vi "Sensor_Reads.vi"() -> ()   [LabVIEW 2019]
uses:
  M14 Hardware/Flywheel/M14_Flywheel_Hardware_Globals.vi
  <vilib>/Rock Robotics/WPI/ThirdParty/Phoenix-LabVIEW/Motor Controller/Get/CTRE_Phoenix_MotorController_GetSelectedSensorData.vi
  Sensor_Values.vi
  M14 Hardware/Drive/M14_Drive_Hardware_Globals.vi
  M14 Hardware/Spindexer/M14_Hardware_Spindexer_Globals.vi
  M14 Hardware/New Magazine/New_Magazine_Hardware_Globals.vi
  M14 Hardware/Turret/M14 Turret_Hardware_Globals.vi
  M14 Hardware/Control Panel/M14_Control_Panel_Globals.vi
  M14 Hardware/Sensors/IMU/M14_IMU_Hardware_Globals.vi
  M14 Hardware/Sensors/IRs & Limits/M14_IR&Limits_Hardware_Globals.vi
  M14 Hardware/Cowl/M14_Cowl_Hardware_Globals.vi
  <vilib>/Rock Robotics/Network Tables/NT Read Number.vi
  <vilib>/Rock Robotics/WPI/ThirdParty/Phoenix-LabVIEW/Pigeon IMU/CTRE_PigeonIMU_GetYPR.vi
panel:
  in  "ball_detected_threshold(ms)":u32
  out "Y_Position(Feet)":dbl
  out "X_Position(Feet)":dbl
  out "Right_Drive_Position(feet)":dbl
  out "Left_Drive_Position(feet)":dbl
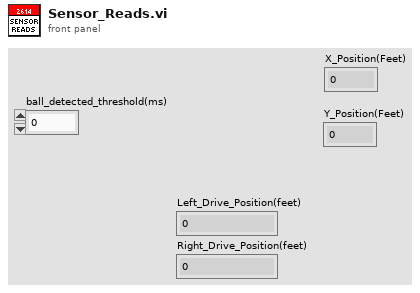
[diagram p1: front panel]
types:
  T1 = typedef "WPI_MotorControlDeviceRef.ctl" = cluster{"DeviceStatus":errorcluster, "Type":T2, "PWM":cluster{"PWM Channel":T3, "DeadBand":T4}, "CAN":cluster{"Device Number":u8, "SetOutput VI Ref":variant, "GetOutput VI Ref":variant, "Enable VI Ref":variant, "Disable VI Ref":variant, "Data":variant}, "Invert":bool, "DIO PWM":cluster{"PWM \"Enable\" Channel":T3, "DIOChannel":T5, "PWM Rate":dbl}}
  T2 = typedef "WPI_MotorControlType.ctl" = enum16{"PWM", "CAN", "DIO PWM"}
  T3 = typedef "FPGA_DIOPWMChannel.ctl" = enum8{"PWM 0", "PWM 1", "PWM 2", "PWM 3", "PWM 4", "PWM 5", "PWM 6", "PWM 7", "PWM 8", "PWM 9", "PWM MXP 0", "PWM MXP 1", "PWM MXP 2", "PWM MXP 3", "PWM MXP 4", "PWM MXP 5", "PWM MXP 6", "PWM MXP 7", "PWM MXP 8", "PWM MXP 9", "Invalid"}
  T4 = typedef "WPI_PWMDeadband.ctl" = cluster{"Name":string, "maxPositivePwm":i32, "minPositivePwm":i32, "centerPwm":i32, "maxNegativePwm":i32, "minNegativePwm":i32, "angularRange":u16}
  T5 = typedef "FPGA_DIOChannel.ctl" = enum8{"DIO 0", "DIO 1", "DIO 2", "DIO 3", "DIO 4", "DIO 5", "DIO 6", "DIO 7", "DIO 8", "DIO 9", "DIO MXP 0", "DIO MXP 1", "DIO MXP 2", "DIO MXP 3", "DIO MXP 4", "DIO MXP 5", "DIO MXP 6", "DIO MXP 7", "DIO MXP 8", "DIO MXP 9", "DIO MXP 10", "DIO MXP 11", "DIO MXP 12", "DIO MXP 13", "DIO MXP 14", "DIO MXP 15", "SPI Port CS1", "SPI Port CS2", "SPI Port CS3", "SPI Port MISO", "SPI Port MOSI", "Invalid"}
  T6 = typedef "CTRE_PigeonIMU_DeviceRef.ctl" = cluster{"DeviceStatus":errorcluster, "Device Number":u8, "Type":T7, "Device ID":u32, "Handle":u64, "UsageFrame":u32, "Library Path":path}
  T7 = typedef "CTRE_PigeonIMU_ConnectionType.ctl" = u32
  T8 = typedef "WPI_DigitalInputDevRef.ctl" = cluster{"DevStatus":errorcluster, "DIO Channel":T5}
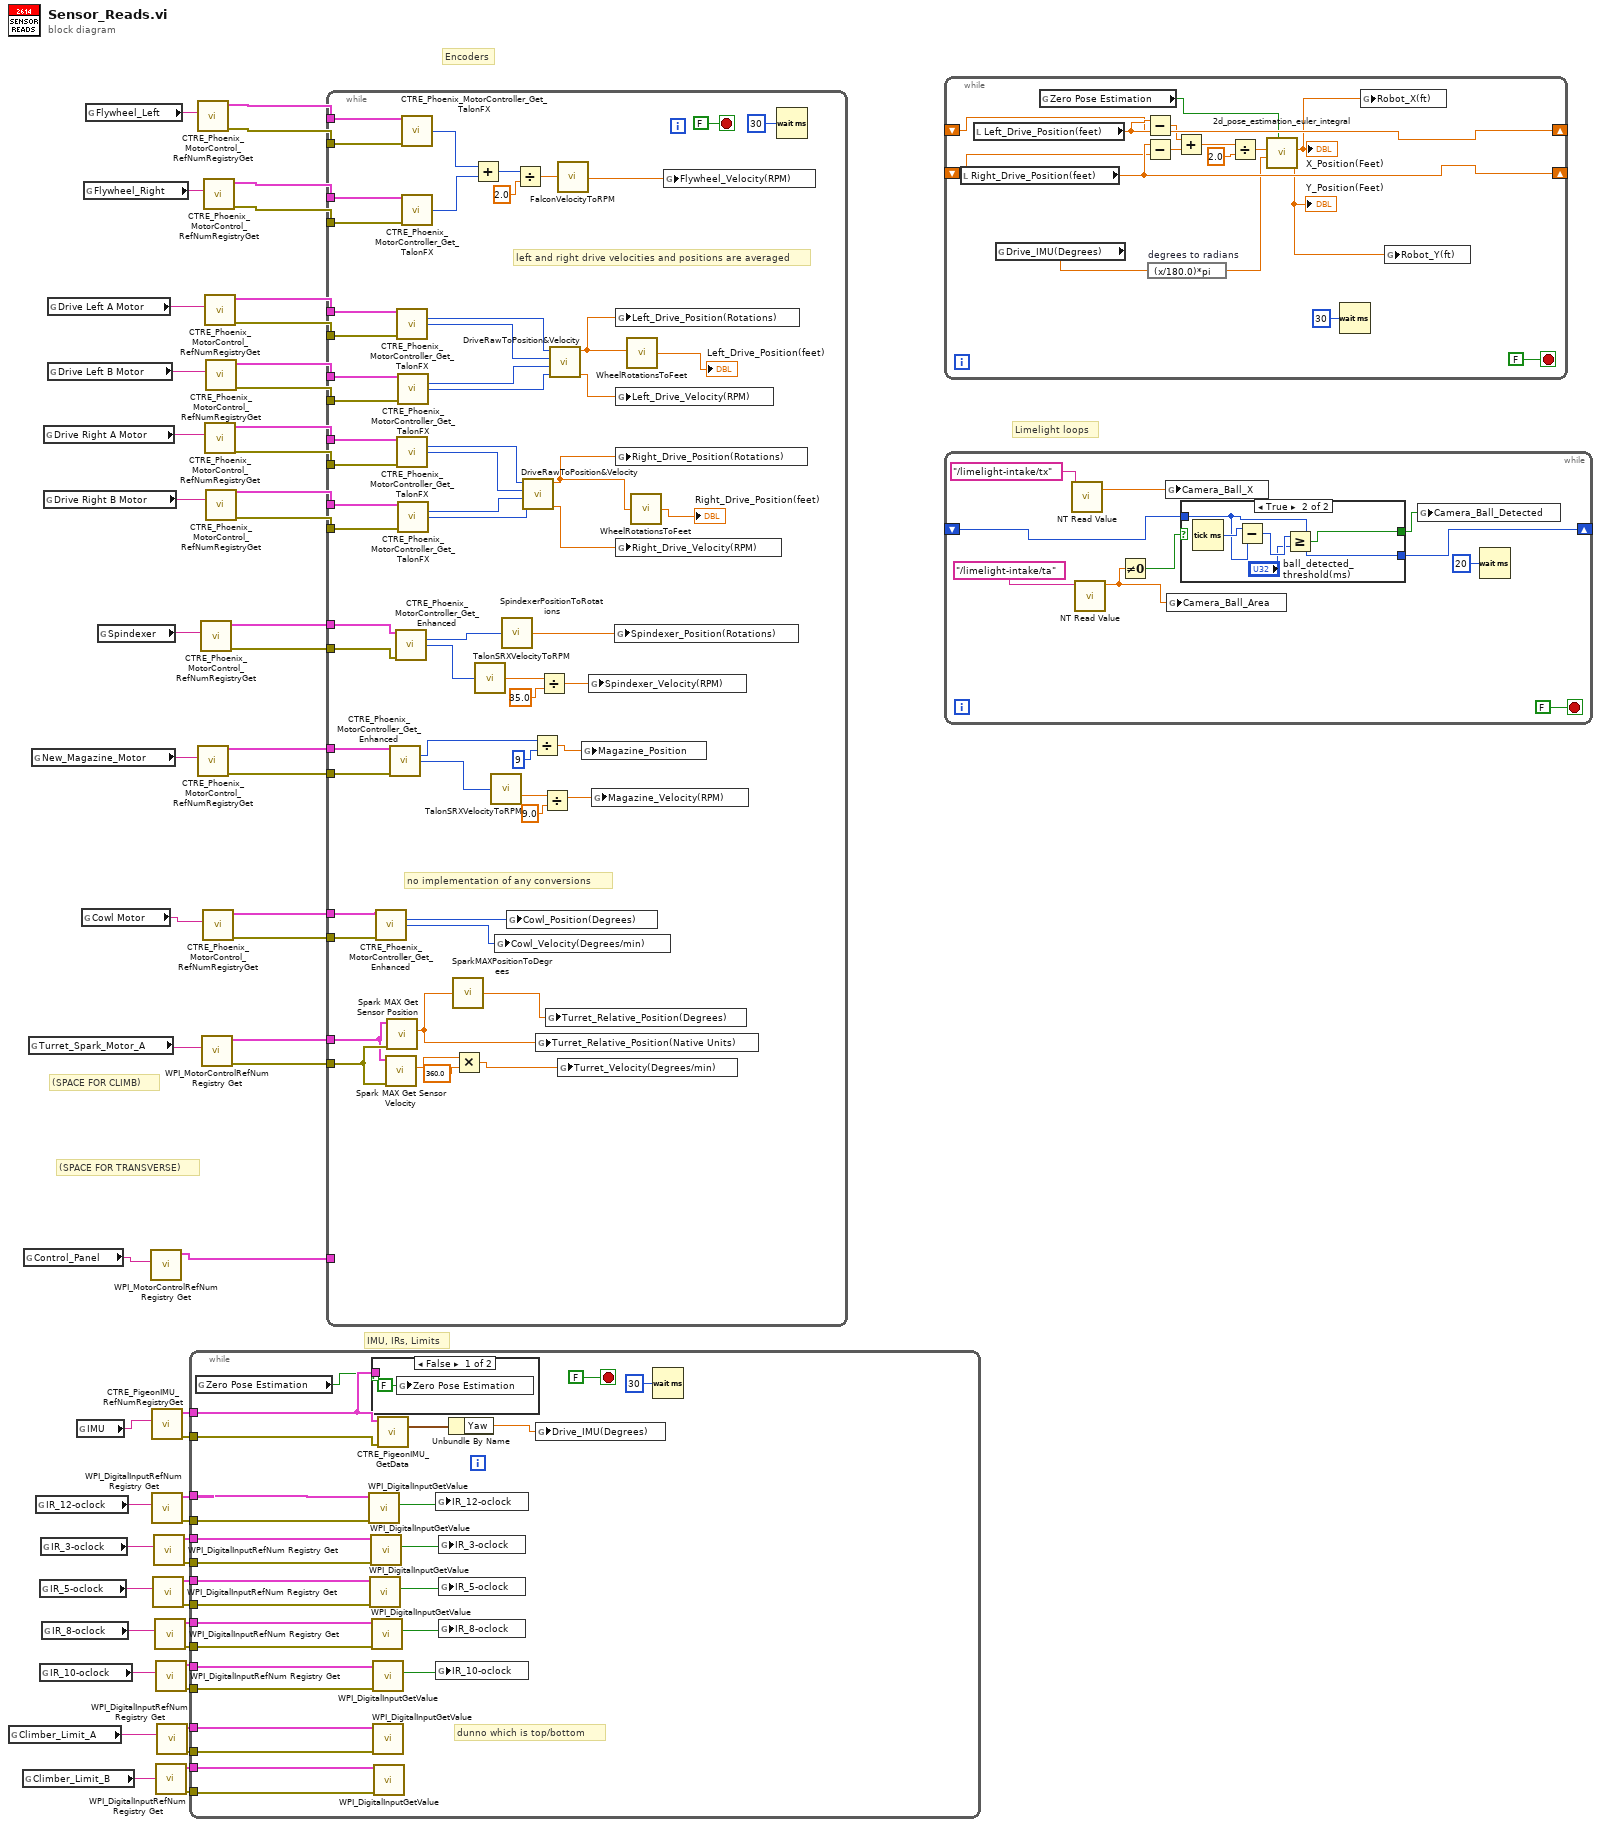
[diagram p0: block diagram]
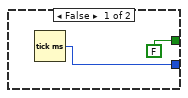
[diagram p2: hidden frame]
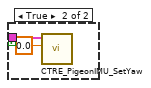
[diagram p3: hidden frame]
diagram:
  # "Limelight loops"
  # "IMU, IRs, Limits"
  # "(SPACE FOR TRANSVERSE)"
  # "(SPACE FOR CLIMB)"
  # "Encoders"
  n1 = global read "M14_IR&Limits_Hardware_Globals.vi" "Climber_Limit_A"() -> (w9:string)
  n2 = global read "M14_IR&Limits_Hardware_Globals.vi" "Climber_Limit_B"() -> (w8:string)
  n3 = global read "M14_Control_Panel_Globals.vi" "Control_Panel"() -> (w36:string)
  n4 = global read "M14 Turret_Hardware_Globals.vi" "Turret_Spark_Motor_A"() -> (w38:string)
  n5 = global read "New_Magazine_Hardware_Globals.vi" "New_Magazine_Motor"() -> (w40:string)
  n6 = global read "M14_IR&Limits_Hardware_Globals.vi" "IR_12-oclock"() -> (w22:string)
  n7 = global read "M14_IR&Limits_Hardware_Globals.vi" "IR_5-oclock"() -> (w16:string)
  n8 = global read "M14_IR&Limits_Hardware_Globals.vi" "IR_10-oclock"() -> (w10:string)
  n9 = global read "M14_IR&Limits_Hardware_Globals.vi" "IR_3-oclock"() -> (w21:string)
  n10 = global read "M14_IR&Limits_Hardware_Globals.vi" "IR_8-oclock"() -> (w15:string)
  n11 = global read "M14_Drive_Hardware_Globals.vi" "Drive Right A Motor"() -> (w43:string)
  n12 = global read "M14_Drive_Hardware_Globals.vi" "Drive Right B Motor"() -> (w46:string)
  n13 = global read "M14_Drive_Hardware_Globals.vi" "Drive Left A Motor"() -> (w50:string)
  n14 = global read "M14_Drive_Hardware_Globals.vi" "Drive Left B Motor"() -> (w47:string)
  n15 = global read "M14_IMU_Hardware_Globals.vi" "IMU"() -> (w34:string)
  n16 = global read "M14_Cowl_Hardware_Globals.vi" "Cowl Motor"() -> (w3:string)
  n17 = global read "M14_Flywheel_Hardware_Globals.vi" "Flywheel_Right"() -> (w55:string)
  n18 = global read "M14_Flywheel_Hardware_Globals.vi" "Flywheel_Left"() -> (w56:string)
  n19 = global read "M14_Hardware_Spindexer_Globals.vi" "Spindexer"() -> (w42:string)
  n20 = call <vilib>:"WPI_MotorControlRefNum Registry Get.vi"("refnum name"=w36) -> ("MotorControlDevRef"=w35:T1)  [unwired: 9 in, 1 out]
  n21 = call <vilib>:"CTRE_PigeonIMU_RefNumRegistryGet.vi"("refnum name"=w34) -> ("error out"=w25:errorcluster, "PigeonIMUDevRef"=w33:T6)  [unwired: 9 in]
  n22 = call <vilib>:"WPI_DigitalInputRefNum Registry Get.vi"("refnum name"=w22) -> ("error out"=w23:errorcluster, "DigitalInputDevRef"=w24:T8)  [unwired: 9 in]
  n23 = call <vilib>:"WPI_DigitalInputRefNum Registry Get.vi"("refnum name"=w16) -> ("error out"=w17:errorcluster, "DigitalInputDevRef"=w18:T8)  [unwired: 9 in]
  n24 = call <vilib>:"WPI_DigitalInputRefNum Registry Get.vi"("refnum name"=w21) -> ("error out"=w20:errorcluster, "DigitalInputDevRef"=w19:T8)  [unwired: 9 in]
  n25 = call <vilib>:"WPI_DigitalInputRefNum Registry Get.vi"("refnum name"=w15) -> ("error out"=w14:errorcluster, "DigitalInputDevRef"=w13:T8)  [unwired: 9 in]
  n26 = call <vilib>:"WPI_DigitalInputRefNum Registry Get.vi"("refnum name"=w10) -> ("error out"=w11:errorcluster, "DigitalInputDevRef"=w12:T8)  [unwired: 9 in]
  n27 = call <vilib>:"WPI_DigitalInputRefNum Registry Get.vi"("refnum name"=w8) -> ("error out"=w4:errorcluster, "DigitalInputDevRef"=w5:T8)  [unwired: 9 in]
  n28 = call <vilib>:"WPI_DigitalInputRefNum Registry Get.vi"("refnum name"=w9) -> ("error out"=w6:errorcluster, "DigitalInputDevRef"=w7:T8)  [unwired: 9 in]
  n29 = while {
    tunnel: w33 -> [w58]
    tunnel: w25 -> [w81]
    tunnel: w24 -> [w78]
    tunnel: w23 -> [w77]
    tunnel: w19 -> [w75]
    tunnel: w20 -> [w76]
    tunnel: w18 -> [w74]
    tunnel: w17 -> [w73]
    tunnel: w13 -> [w71]
    tunnel: w14 -> [w72]
    tunnel: w12 -> [w70]
    tunnel: w11 -> [w69]
    tunnel: w7 -> [w63]
    tunnel: w6 -> [w62]
    tunnel: w5 -> [w61]
    tunnel: w4 -> [w60]
    stop <- FALSE stop-if-true
    # "dunno which is top/bottom"
    n30 = global read "Sensor_Values.vi" "Zero Pose Estimation"() -> (w57:bool)
    n31 = call <vilib>:"WPI_DigitalInputGetValue.vi"("error in (no error)"=w77, "DigitalInputDevRef"=w78) -> ("Value"=w68:bool)  [unwired: 7 in, 2 out]
    n32 = call <vilib>:"WPI_DigitalInputGetValue.vi"("error in (no error)"=w73, "DigitalInputDevRef"=w74) -> ("Value"=w66:bool)  [unwired: 7 in, 2 out]
    n33 = call <vilib>:"WPI_DigitalInputGetValue.vi"("error in (no error)"=w76, "DigitalInputDevRef"=w75) -> ("Value"=w67:bool)  [unwired: 7 in, 2 out]
    n34 = case shown="False" w57 {
      tunnel: w58 -> [_ w85]
      frame False {
        n35 = global write "Sensor_Values.vi" "Zero Pose Estimation"(FALSE ("Zero Pose Estimation")) -> ()
      }
      frame True {
        n36 = call <vilib>:"CTRE_PigeonIMU_SetYaw.vi"("Value"=0.0, "PigeonIMUDevRef"=w85) -> ()  [unwired: 8 in, 2 out]
      }
    }
    n37 = call <vilib>:"WPI_DigitalInputGetValue.vi"("error in (no error)"=w72, "DigitalInputDevRef"=w71) -> ("Value"=w65:bool)  [unwired: 7 in, 2 out]
    n38 = call <vilib>:"WPI_DigitalInputGetValue.vi"("error in (no error)"=w69, "DigitalInputDevRef"=w70) -> ("Value"=w64:bool)  [unwired: 7 in, 2 out]
    n39 = call <vilib>:"WPI_DigitalInputGetValue.vi"("error in (no error)"=w62, "DigitalInputDevRef"=w63) -> ()  [unwired: 7 in, 3 out]
    n40 = call <vilib>:"WPI_DigitalInputGetValue.vi"("error in (no error)"=w60, "DigitalInputDevRef"=w61) -> ()  [unwired: 7 in, 3 out]
    n41 = call-poly <vilib>:"CTRE_PigeonIMU_GetData.vi"("error in (no error)"=w81, "PigeonIMUDevRef"=w58) -> ("Yaw Pitch Roll"=w80:cluster{"Yaw":dbl, "Pitch":dbl, "Roll":dbl})  [unwired: 7 in, 2 out]
    n42 = global write "Sensor_Values.vi" "IR_12-oclock"(w68) -> ()
    n43 = global write "Sensor_Values.vi" "IR_10-oclock"(w64) -> ()
    n44 = global write "Sensor_Values.vi" "IR_3-oclock"(w67) -> ()
    n45 = global write "Sensor_Values.vi" "IR_5-oclock"(w66) -> ()
    n46 = global write "Sensor_Values.vi" "IR_8-oclock"(w65) -> ()
    n47 = Unbundle By Name(w80) -> ("Yaw"=w59:dbl)
    n48 = global write "Sensor_Values.vi" "Drive_IMU(Degrees)"(w59) -> ()
    n49 = Wait (ms)(milliseconds to wait=u32 30) -> ()  [unwired: 1 out]
  }
  n50 = call <vilib>:"CTRE_Phoenix_MotorControl_RefNumRegistryGet.vi"("refnum name"=w56) -> ("error out"=w53:errorcluster, "PhoenixMotorControlDevRef"=w54:T1)  [unwired: 9 in]
  n51 = call <vilib>:"CTRE_Phoenix_MotorControl_RefNumRegistryGet.vi"("refnum name"=w40) -> ("error out"=w27:errorcluster, "PhoenixMotorControlDevRef"=w39:T1)  [unwired: 9 in]
  n52 = call <vilib>:"CTRE_Phoenix_MotorControl_RefNumRegistryGet.vi"("refnum name"=w42) -> ("error out"=w28:errorcluster, "PhoenixMotorControlDevRef"=w41:T1)  [unwired: 9 in]
  n53 = call <vilib>:"WPI_MotorControlRefNum Registry Get.vi"("refnum name"=w38) -> ("error out"=w26:errorcluster, "MotorControlDevRef"=w37:T1)  [unwired: 9 in]
  n54 = call <vilib>:"CTRE_Phoenix_MotorControl_RefNumRegistryGet.vi"("refnum name"=w3) -> ("error out"=w1:errorcluster, "PhoenixMotorControlDevRef"=w2:T1)  [unwired: 9 in]
  n55 = call <vilib>:"CTRE_Phoenix_MotorControl_RefNumRegistryGet.vi"("refnum name"=w55) -> ("error out"=w51:errorcluster, "PhoenixMotorControlDevRef"=w52:T1)  [unwired: 9 in]
  n56 = call <vilib>:"CTRE_Phoenix_MotorControl_RefNumRegistryGet.vi"("refnum name"=w50) -> ("error out"=w32:errorcluster, "PhoenixMotorControlDevRef"=w49:T1)  [unwired: 9 in]
  n57 = call <vilib>:"CTRE_Phoenix_MotorControl_RefNumRegistryGet.vi"("refnum name"=w43) -> ("error out"=w30:errorcluster, "PhoenixMotorControlDevRef"=w44:T1)  [unwired: 9 in]
  n58 = call <vilib>:"CTRE_Phoenix_MotorControl_RefNumRegistryGet.vi"("refnum name"=w47) -> ("error out"=w31:errorcluster, "PhoenixMotorControlDevRef"=w48:T1)  [unwired: 9 in]
  n59 = call <vilib>:"CTRE_Phoenix_MotorControl_RefNumRegistryGet.vi"("refnum name"=w46) -> ("error out"=w29:errorcluster, "PhoenixMotorControlDevRef"=w45:T1)  [unwired: 9 in]
  n60 = while {
    tunnel: w54 -> [w145]
    tunnel: w53 -> [w144]
    tunnel: w52 -> [w143]
    tunnel: w51 -> [w142]
    tunnel: w49 -> [w141]
    tunnel: w48 -> [w140]
    tunnel: w44 -> [w138]
    tunnel: w45 -> [w139]
    tunnel: w41 -> [w128]
    tunnel: w39 -> [w125]
    tunnel: w37 -> [w106]
    tunnel: w35 -> [_]
    tunnel: w32 -> [w113]
    tunnel: w31 -> [w112]
    tunnel: w30 -> [w111]
    tunnel: w29 -> [w110]
    tunnel: w28 -> [w109]
    tunnel: w27 -> [w108]
    tunnel: w26 -> [w107]
    tunnel: w2 -> [w89]
    tunnel: w1 -> [w88]
    stop <- FALSE stop-if-true
    # "no implementation of any conversions"
    # "left and right drive velocities and positions are averaged"
    n61 = call-poly <vilib>:"CTRE_Phoenix_MotorController_Get_Enhanced.vi"("PhoenixMotorControlDevRef"=w89, "error in"=w88) -> ("Position (Raw Sensor Units)"=w87:i32, "Velocity (Raw Sensor Units per 100 ms)"=w86:i32)  [unwired: 10 in, 2 out]
    n62 = call <vilib>:"Spark MAX Get Sensor Velocity.vi"("error in (no error)"=w107, "MotorControlDevRef in"=w106) -> ("Sensor Velocity"=w97:dbl)  [unwired: 6 in, 3 out]
    n63 = call <vilib>:"Spark MAX Get Sensor Position.vi"("error in (no error)"=w107, "MotorControlDevRef in"=w106) -> ("Sensor Position"=w94:dbl)  [unwired: 6 in, 3 out]
    n64 = call-poly <vilib>:"CTRE_Phoenix_MotorController_Get_Enhanced.vi"("PhoenixMotorControlDevRef"=w125, "error in"=w108) -> ("Position (Raw Sensor Units)"=w121:i32, "Velocity (Raw Sensor Units per 100 ms)"=w124:i32)  [unwired: 10 in, 2 out]
    n65 = call-poly <vilib>:"CTRE_Phoenix_MotorController_Get_Enhanced.vi"("PhoenixMotorControlDevRef"=w128, "error in"=w109) -> ("Position (Raw Sensor Units)"=w126:i32, "Velocity (Raw Sensor Units per 100 ms)"=w127:i32)  [unwired: 10 in, 2 out]
    n66 = call-poly <vilib>:"CTRE_Phoenix_MotorController_Get_TalonFX.vi"("PhoenixMotorControlDevRef"=w141, "error in"=w113) -> ("Position (Raw Sensor Units)"=w130:i32, "Velocity (Raw Sensor Units per 100 ms)"=w137:i32)  [unwired: 10 in, 2 out]
    n67 = call-poly <vilib>:"CTRE_Phoenix_MotorController_Get_TalonFX.vi"("PhoenixMotorControlDevRef"=w138, "error in"=w111) -> ("Position (Raw Sensor Units)"=w103:i32, "Velocity (Raw Sensor Units per 100 ms)"=w102:i32)  [unwired: 10 in, 2 out]
    n68 = call-poly <vilib>:"CTRE_Phoenix_MotorController_Get_TalonFX.vi"("PhoenixMotorControlDevRef"=w140, "error in"=w112) -> ("Position (Raw Sensor Units)"=w129:i32, "Velocity (Raw Sensor Units per 100 ms)"=w105:i32)  [unwired: 10 in, 2 out]
    n69 = call-poly <vilib>:"CTRE_Phoenix_MotorController_Get_TalonFX.vi"("PhoenixMotorControlDevRef"=w139, "error in"=w110) -> ("Position (Raw Sensor Units)"=w101:i32, "Velocity (Raw Sensor Units per 100 ms)"=w100:i32)  [unwired: 10 in, 2 out]
    n70 = call-poly <vilib>:"CTRE_Phoenix_MotorController_Get_TalonFX.vi"("PhoenixMotorControlDevRef"=w145, "error in"=w144) -> ("Velocity (Raw Sensor Units per 100 ms)"=w133:i32)  [unwired: 10 in, 3 out]
    n71 = call-poly <vilib>:"CTRE_Phoenix_MotorController_Get_TalonFX.vi"("PhoenixMotorControlDevRef"=w143, "error in"=w142) -> ("Velocity (Raw Sensor Units per 100 ms)"=w132:i32)  [unwired: 10 in, 3 out]
    n72 = call "SparkMAXPositionToDegrees.vi"("Sensor Position"=w94) -> ("degrees"=w95:dbl)  [unwired: 4 in]
    n73 = Multiply(x=w97, y=360.0) -> (x*y=w98:dbl)
    n74 = Add(x=w133, y=w132) -> (x+y=w134:i32)
    n75 = call "TalonSRXVelocityToRPM.vi"("Velocity (Raw Sensor Units per 100 ms)"=w127) -> ("RPM"=w117:dbl)  [unwired: 4 in]
    n76 = call "TalonSRXVelocityToRPM.vi"("Velocity (Raw Sensor Units per 100 ms)"=w124) -> ("RPM"=w123:dbl)  [unwired: 4 in]
    n77 = global write "Sensor_Values.vi" "Cowl_Velocity(Degrees/min)"(w86) -> ()
    n78 = call "SpindexerPositionToRotations.vi"("Position (Raw Sensor Units)"=w126) -> ("Numeric"=w114:dbl)  [unwired: 4 in]
    n79 = global write "Sensor_Values.vi" "Cowl_Position(Degrees)"(w87) -> ()
    n80 = Divide(x=w134, y=2.0) -> (x/y=w131:dbl)
    n81 = call "DriveRawToPosition&Velocity.vi"("Velocity (Raw Sensor Units per 100 ms) B"=w100, "Position (Raw Sensor Units) B"=w101, "Velocity (Raw Sensor Units per 100 ms) A"=w102, "Position (Raw Sensor Units) A"=w103) -> ("Velocity"=w99:dbl, "Position"=w91:dbl)  [unwired: 6 in]
    n82 = Divide(x=w121, y=9) -> (x/y=w122:dbl)
    n83 = global write "Sensor_Values.vi" "Turret_Relative_Position(Native Units)"(w94) -> ()
    n84 = Divide(x=w117, y=35.0) -> (x/y=w115:dbl)
    n85 = Divide(x=w123, y=9.0) -> (x/y=w119:dbl)
    n86 = global write "Sensor_Values.vi" "Turret_Relative_Position(Degrees)"(w95) -> ()
    n87 = call "DriveRawToPosition&Velocity.vi"("Velocity (Raw Sensor Units per 100 ms) B"=w105, "Position (Raw Sensor Units) B"=w129, "Velocity (Raw Sensor Units per 100 ms) A"=w137, "Position (Raw Sensor Units) A"=w130) -> ("Velocity"=w104:dbl, "Position"=w93:dbl)  [unwired: 6 in]
    n88 = call "FalconVelocityToRPM.vi"("raw sensor units / 100 ms"=w131) -> ("RPM"=w136:dbl)  [unwired: 4 in]
    n89 = global write "Sensor_Values.vi" "Turret_Velocity(Degrees/min)"(w98) -> ()
    n90 = global write "Sensor_Values.vi" "Magazine_Position"(w122) -> ()
    n91 = global write "Sensor_Values.vi" "Spindexer_Velocity(RPM)"(w115) -> ()
    n92 = global write "Sensor_Values.vi" "Magazine_Velocity(RPM)"(w119) -> ()
    n93 = global write "Sensor_Values.vi" "Spindexer_Position(Rotations)"(w114) -> ()
    n94 = global write "Sensor_Values.vi" "Left_Drive_Position(Rotations)"(w93) -> ()
    n95 = global write "Sensor_Values.vi" "Left_Drive_Velocity(RPM)"(w104) -> ()
    n96 = global write "Sensor_Values.vi" "Right_Drive_Position(Rotations)"(w91) -> ()
    n97 = global write "Sensor_Values.vi" "Right_Drive_Velocity(RPM)"(w99) -> ()
    n98 = call "WheelRotationsToFeet.vi"("rotations"=w93) -> ("feet"=→"Left_Drive_Position(feet)":dbl)  [unwired: 4 in]
    n99 = call "WheelRotationsToFeet.vi"("rotations"=w91) -> ("feet"=→"Right_Drive_Position(feet)":dbl)  [unwired: 4 in]
    n100 = global write "Sensor_Values.vi" "Flywheel_Velocity(RPM)"(w136) -> ()
    n101 = Wait (ms)(milliseconds to wait=u32 30) -> ()  [unwired: 1 out]
  }
  n102 = while {
    shift-right: [w163] -> _
    shift-left: _ -> [w162]
    shift-right: [w161] -> _
    shift-left: _ -> [w160]
    stop <- FALSE stop-if-true
    n103 = local read "Right_Drive_Position(feet)"() -> (w161:dbl)
    n104 = local read "Left_Drive_Position(feet)"() -> (w163:dbl)
    n105 = global read "Sensor_Values.vi" "Drive_IMU(Degrees)"() -> (w154:dbl)
    n106 = global read "Sensor_Values.vi" "Zero Pose Estimation"() -> (w148:bool)
    n107 = Subtract(x=w163, y=w162) -> (x-y=w159:dbl)
    n108 = Subtract(x=w161, y=w160) -> (x-y=w158:dbl)
    n109 = expression code="(x/180.0)*pi" "degrees to radians"(w154) -> (w153:dbl)
    n110 = Add(x=w159, y=w158) -> (x+y=w157:dbl)
    n111 = Divide(x=w157, y=2.0) -> (x/y=w155:dbl)
    n112 = call "2d_pose_estimation_euler_integral.vi"("Zero XY?"=w148, "theta(rad)"=w153, "v(per tick)"=w155) -> ("y"=w150:dbl, "x"=w151:dbl)  [unwired: 7 in]
    "X_Position(Feet)" <- w151
    "Y_Position(Feet)" <- w150
    n113 = Wait (ms)(milliseconds to wait=u32 30) -> ()  [unwired: 1 out]
    n114 = global write "Sensor_Values.vi" "Robot_X(ft)"(w151) -> ()
    n115 = global write "Sensor_Values.vi" "Robot_Y(ft)"(w150) -> ()
  }
  n116 = while {
    shift-right: [w165] -> _
    shift-left: _ -> [w164]
    stop <- FALSE stop-if-true
    n117 = call-poly <vilib>:"NT Read Value.vi"("Name"="/limelight-intake/tx") -> ("Numeric"=w170:dbl)  [unwired: 9 in, 1 out]
    n118 = call-poly <vilib>:"NT Read Value.vi"("Name"="/limelight-intake/ta") -> ("Numeric"=w169:dbl)  [unwired: 9 in, 1 out]
    n119 = Not Equal To 0?(x=w169) -> (x != 0?=w167:bool)
    n120 = global write "Sensor_Values.vi" "Camera_Ball_X"(w170) -> ()
    n121 = global write "Sensor_Values.vi" "Camera_Ball_Area"(w169) -> ()
    n122 = case shown="True" w167 {
      tunnel: [FALSE ("Camera_Ball_Detected") w180] -> w166
      tunnel: [w174 w178] -> w165
      tunnel: w164 -> [_ w178]
      frame False {
        n123 = Tick Count (ms)() -> (millisecond timer value=w174:u32)
      }
      frame True {
        n124 = Tick Count (ms)() -> (millisecond timer value=w179:u32)
        n125 = Subtract(x=w179, y=w178) -> (x-y=w177:u32)
        n126 = Greater Or Equal?(x=w177, y="ball_detected_threshold(ms)") -> (x >= y?=w180:bool)
      }
    }
    n127 = global write "Sensor_Values.vi" "Camera_Ball_Detected"(w166) -> ()
    n128 = Wait (ms)(milliseconds to wait=u32 20) -> ()  [unwired: 1 out]
  }
